vi "Configure_Voltage.vi"(6 "Measurement Type":T2(ring), 8 "error in (no error)":errorcluster, 9 "Resolution in Digits":T1(ring), 10 "Range":dbl=1.2, 11 "NI-DCPower in":refnum<class "niDCPower.lvclass">) -> (0 "error out":errorcluster, 3 "NI-DCpower out":refnum<class "niDCPower.lvclass">)   [LabVIEW 2021, in "niDCPower.lvclass"]
uses:
  niDCPower.lvclass
  <instrlib>/niDCPower/nidcpower.llb/niDCPower Source Mode.ctl
  niDCPower.lvclass/niDCPower.ctl
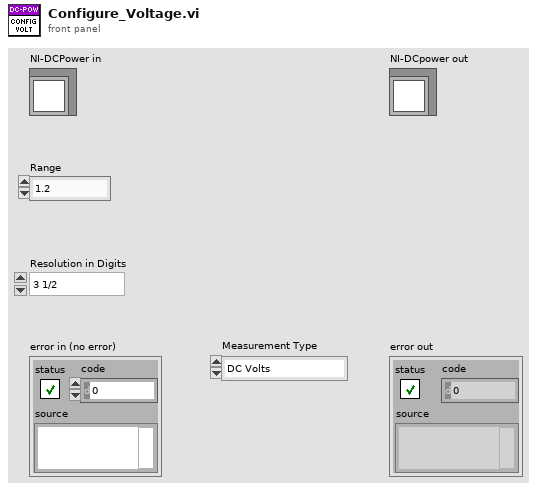
[diagram p1: front panel]
types:
  T1 = enum32{"3 1/2", "4 1/2", "5 1/2", "6 1/2", "7 1/2"}
  T2 = enum32{"DC Volts", "AC Volts", "DC Current", "AC Current", "2-wire Resistance", "4-wire Resistance", "Diode", "Frequency", "Period", "AC Volts DC Coupled", "Capacitance", "Inductance", "Temperature"}
  T3 = typedef "niDCPower Source Mode.ctl" = i32
  T4 = typedef "niDCPower Output Function.ctl" = i32
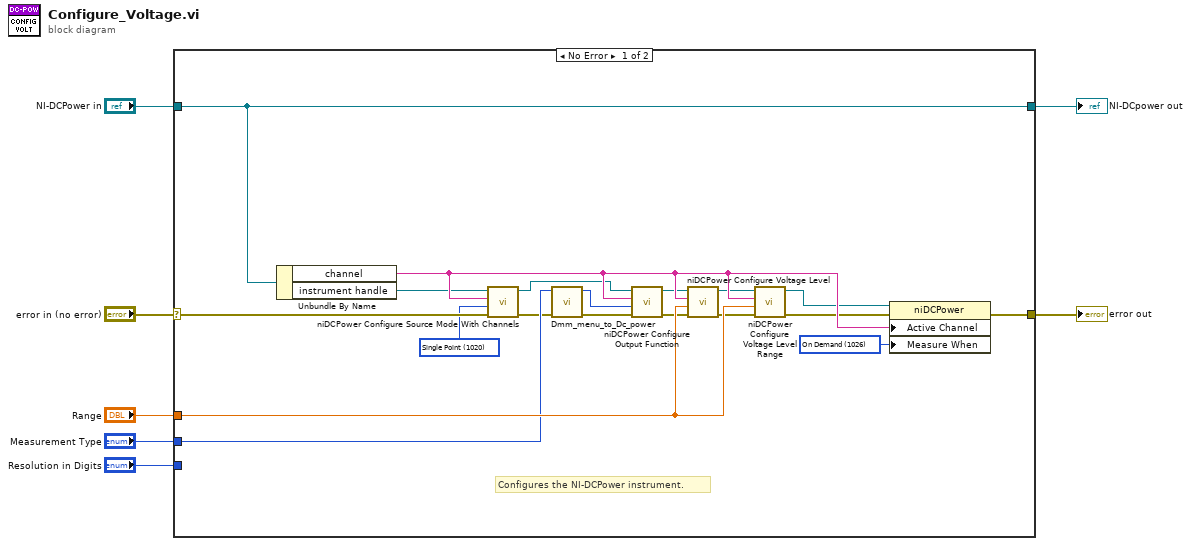
[diagram p0: block diagram]
diagram:
  n1 = case shown="No Error" "error in (no error)" {
    selector: "error in (no error)" -> [w26 w27]
    tunnel: [w25 w27] -> w6
    tunnel: "NI-DCPower in" -> [w22 w28]
    tunnel: [w22 w28] -> w4
    tunnel: "Range" -> [w24 _]
    tunnel: "Measurement Type" -> [w23 _]
    tunnel: "Resolution in Digits" -> [_ _]
    frame No Error {
      w11 = 1026 items=["Automatically after Source Complete"=1025, "On Demand"=1026, "On Measure Trigger"=1027] ("Measurement:Advanced:Measure When")
      w12 = T3 1020 items=["Single Point"=1020, "Sequence"=1021] ("source mode")
      # "Configures the NI-DCPower instrument."
      n2 = Unbundle By Name(w22) -> ("channel"=w21:string, "instrument handle"=w20:refnum<k15>)
      n3 = call <instrlib>:"niDCPower Configure Source Mode With Channels.vi"("error in (no error)"=w26, "source mode"=w12, "channel name"=w21, "instrument handle"=w20) -> ("error out"=w9:errorcluster, "instrument handle out"=w17:refnum<k15>)  [unwired: 6 in]
      n4 = call "Dmm_menu_to_Dc_power.vi"("error in (no error)"=w9, "Measurement Type"=w23) -> ("error out"=w8:errorcluster, "output function"=w10:T4)  [unwired: 8 in]
      n5 = call <instrlib>:"niDCPower Configure Output Function.vi"("error in (no error)"=w8, "output function"=w10, "channel name"=w21, "instrument handle"=w17) -> ("error out"=w13:errorcluster, "instrument handle out"=w14:refnum<k15>)  [unwired: 6 out]
      n6 = call <instrlib>:"niDCPower Configure Voltage Level.vi"("error in (no error)"=w13, "voltage level"=w24, "channel name"=w21, "instrument handle"=w14) -> ("error out"=w18:errorcluster, "instrument handle out"=w19:refnum<k15>)  [unwired: 6 out]
      n7 = call <instrlib>:"niDCPower Configure Voltage Level Range.vi"("error in (no error)"=w18, "voltage level range"=w24, "channel name"=w21, "instrument handle"=w19) -> ("error out"=w16:errorcluster, "instrument handle out"=w15:refnum<k15>)  [unwired: 6 out]
      n8 = property class="niDCPower"(reference=w15, error in=w16, "Active Channel"=w21, "Measure When"=w11) -> (error out=w25:errorcluster)  [unwired: 1 out]
    }
    frame Error {
    }
  }
  "error out" <- w6
  "NI-DCpower out" <- w4
